vi "2283_lidarPID.vi"(1 "Distance":dbl, 2 "Posicion deseada":dbl format="%.2f") -> (0 "output":dbl format="%.2f")   [LabVIEW 2014]
uses:
  <vilib>/addons/control/pid/pid.llb/PID (DBL).vi
  <vilib>/addons/control/pid/NI_PID_pid.lvlib
panel:
  in  "PID gains":T1
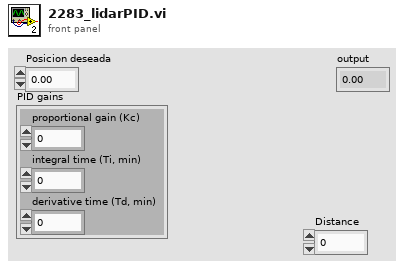
[diagram p1: front panel]
types:
  T1 = cluster{"proportional gain (Kc)":dbl, "integral time (Ti, min)":dbl, "derivative time (Td, min)":dbl}
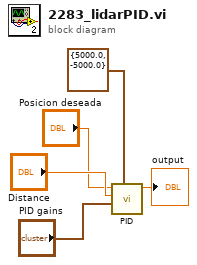
[diagram p0: block diagram]
diagram:
  n1 = call-poly <vilib>:"PID.vi"("output range"=cluster{"output high":dbl, "output low":dbl} {"output high"=5000.0, "output low"=-5000.0}, "PID gains"="PID gains", "process variable"="Distance", "setpoint"="Posicion deseada") -> ("output"=→"output":dbl)  [unwired: 6 in, 1 out]
